vi "ClearID.vi"(0 "G#DebugServer ref":refnum<class "G#Object.lvclass">, 5 "error in (no error)":errorcluster) -> (14 "G#DebugServer ref out":refnum<class "G#Object.lvclass">, 19 "error out":errorcluster)   [LabVIEW 2017, in "G#DebugServer.lvclass"]
doc: "Clears the object ID."
uses:
  <vilib>/addons/_AddQ/G#DebugServer/G#DebugServer.lvclass
  <vilib>/addons/_AddQ/G#Object/G#Object.lvclass
  C:/Program Files (x86)/National Instruments/LabVIEW 2017/vi.lib/addons/_AddQ/G#Object/G#Object.lvclass
  <vilib>/addons/_AddQ/G#DebugServer/G#DebugServer.lvclass/G#DebugServer.ctl
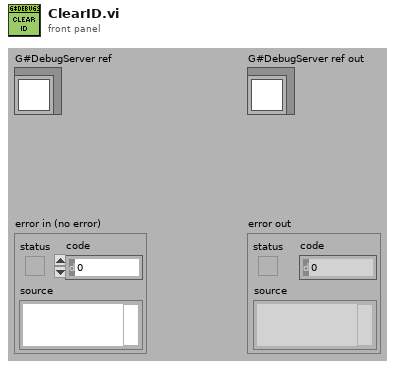
[diagram p1: front panel]
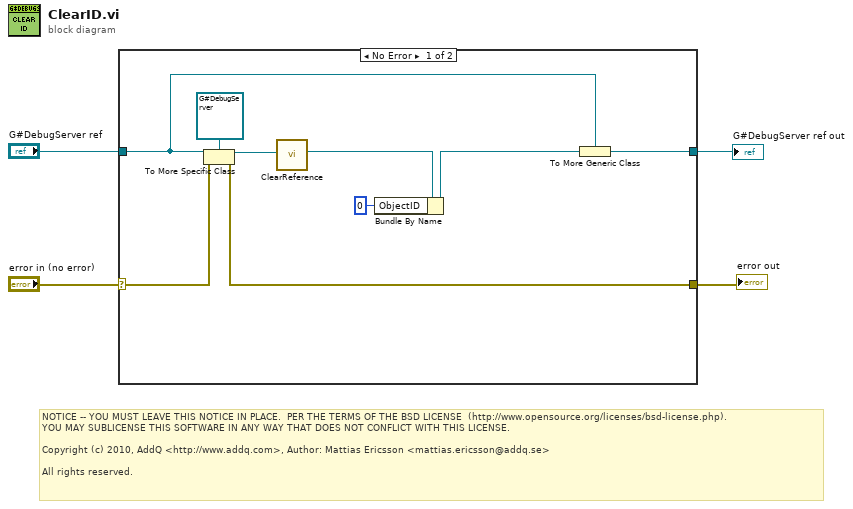
[diagram p0: block diagram]
diagram:
  # "NOTICE -- YOU MUST LEAVE THIS NOTICE IN PLACE.  PER THE TERMS OF THE BSD LICENSE  (http://www.opensource.org/licenses/bsd-license.php).\nYOU MAY SUBLICENSE THIS SOFTWARE IN ANY WAY THAT DOES NOT CONFLICT WITH THIS LICENSE.\n\nCopyright (c) 2010, AddQ <http://www.addq.com>, Author: Mattias Ericsson <mattias.ericsson@addq.se>\n\nAll rights reserved."
  n1 = case shown="No Error" "error in (no error)" {
    selector: "error in (no error)" -> [w13 w15]
    tunnel: [w12 w15] -> w3
    tunnel: "G#DebugServer ref" -> [w6 w14]
    tunnel: [w5 w14] -> w1
    frame No Error {
      n2 = To More Specific Class(target class=refnum<class "G#DebugServer.lvclass"> refnum ("G#DebugServer.lvclass"), reference=w6, error in=w13) -> (specific class reference=w9:refnum<class "G#DebugServer.lvclass">, error out=w12:errorcluster)
      n3 = call-dynamic "ClearReference.vi"("reference in"=w9) -> ("reference out"=w8:refnum<class "G#DebugServer.lvclass">)
      n4 = Bundle By Name(cluster=w8, "ObjectID"=u32 0) -> (w7:refnum<class "G#DebugServer.lvclass">)
      n5 = To More Generic Class(target class=w6, reference=w7) -> (generic class reference=w5:refnum<class "G#Object.lvclass">)
    }
    frame Error {
    }
  }
  "error out" <- w3
  "G#DebugServer ref out" <- w1
